vi "PCO_SetFPSExposureMode.vi"(8 "error in (no error)":errorcluster {"code" format="%x"}, 10 "wFPSExposureMode":u16(ring) items=["OFF", "ON"], 11 "ph":u64) -> (0 "error out":errorcluster {"code" format="%x"}, 1 "dwFPSExposureTime":u32, 2 "ErrorMessage":i32 format="%x", 3 "ph out":u64)   [LabVIEW 2019, in "SDK.lvlib" / "TimingControl.lvlib"]
doc: "<b>Description:</b>\nThis function does set the image timing of the camera so that the maximum frame rate and the maximum exposure time for this frame rate is achieved. The maximum image frame rate (FPS = frames per second) depends on the pixel rate and the image area selection.\n\nIf FPS exposure mode is on other timing commands are ignored.\n\n<b>Supported camera type:</b>\npco.1200\n\n<b>Descriptor dependency:</b>\nNone"
uses:
  TimingControl.lvlib
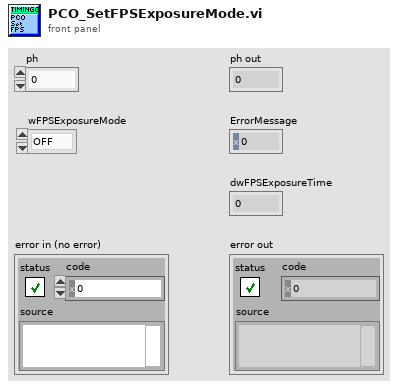
[diagram p1: front panel]
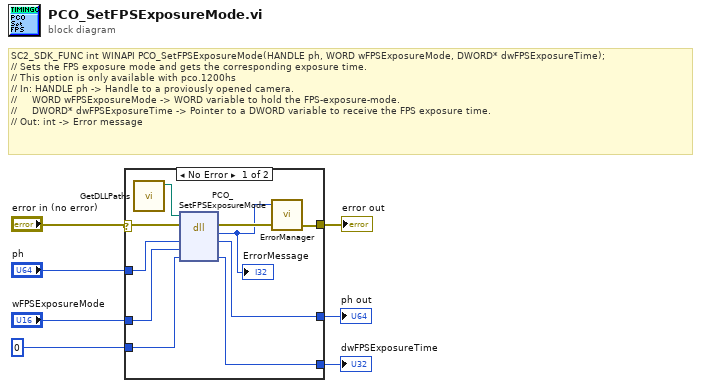
[diagram p0: block diagram]
diagram:
  # "SC2_SDK_FUNC int WINAPI PCO_SetFPSExposureMode(HANDLE ph, WORD wFPSExposureMode, DWORD* dwFPSExposureTime);\n// Sets the FPS exposure mode and gets the corresponding exposure time.\n// This option is only available with pco.1200hs\n// In: HANDLE ph -> Handle to a proviously opened camera.\n//     WORD wFPSExposureMode -> WORD variable to hold the FPS-exposure-mode.\n//     DWORD* dwFPSExposureTime -> Pointer to a DWORD variable to receive the FPS exposure time.\n// Out: int -> Error message"
  n1 = case shown="No Error" "error in (no error)" {
    selector: "error in (no error)" -> [w12 w20]
    tunnel: "ph" -> [w17 w19]
    tunnel: [w16 w19] -> w6
    tunnel: "wFPSExposureMode" -> [w15 _]
    tunnel: u32 0 ("dwFPSExposureTime") -> [w14 w18]
    tunnel: [w13 w18] -> w3
    tunnel: [w10 w20] -> w2
    frame No Error {
      n2 = call "GetDLLPaths.vi"() -> ("SC2_Cam_Path"=w8:path)  [unwired: 8 in, 3 out]
      n3 = dll-call lib="?" fn="PCO_SetFPSExposureMode"(path in=w8, error in=w12, "ph"=w17, "wFPSExposureMode"=w15, "dwFPSExposureTime"=w14) -> (error out=w11:errorcluster, "return type"=w9:i32, "ph"=w16:u64, "dwFPSExposureTime"=w13:u32)  [unwired: 2 in, 1 out]
      "ErrorMessage" <- w9
      n4 = call "ErrorManager.vi"("error in (no error)"=w11, "error code"=w9) -> ("error out"=w10:errorcluster)  [unwired: 2 in, 1 out]
    }
    frame Error {
    }
  }
  "ph out" <- w6
  "dwFPSExposureTime" <- w3
  "error out" <- w2
